vi "Calibrations Control Loop 2017.vi"   [LabVIEW 2016]
uses:
  <vilib>/Rock Robotics/Network Tables/SD Read Boolean.vi
  Global Variables/Ball Intake Calibrations.vi
  Global Variables/Deadband Calibrations.vi
  Global Variables/High Gear Calibrations.vi
  Global Variables/Low Gear Calibrations.vi
  Global Variables/Shooter Calibrations.vi
  Global Variables/Turn to Heading Calibrations.vi
  Global Variables/Drive Path Calibrations.vi
  Global Variables/Conveyor Calibrations.vi
  Global Variables/Auto Drive Calibrations.vi
  <vilib>/Rock Robotics/Network Tables/NT Write Numeric Array.vi
  <vilib>/Rock Robotics/Network Tables/NT Read Numeric Array.vi
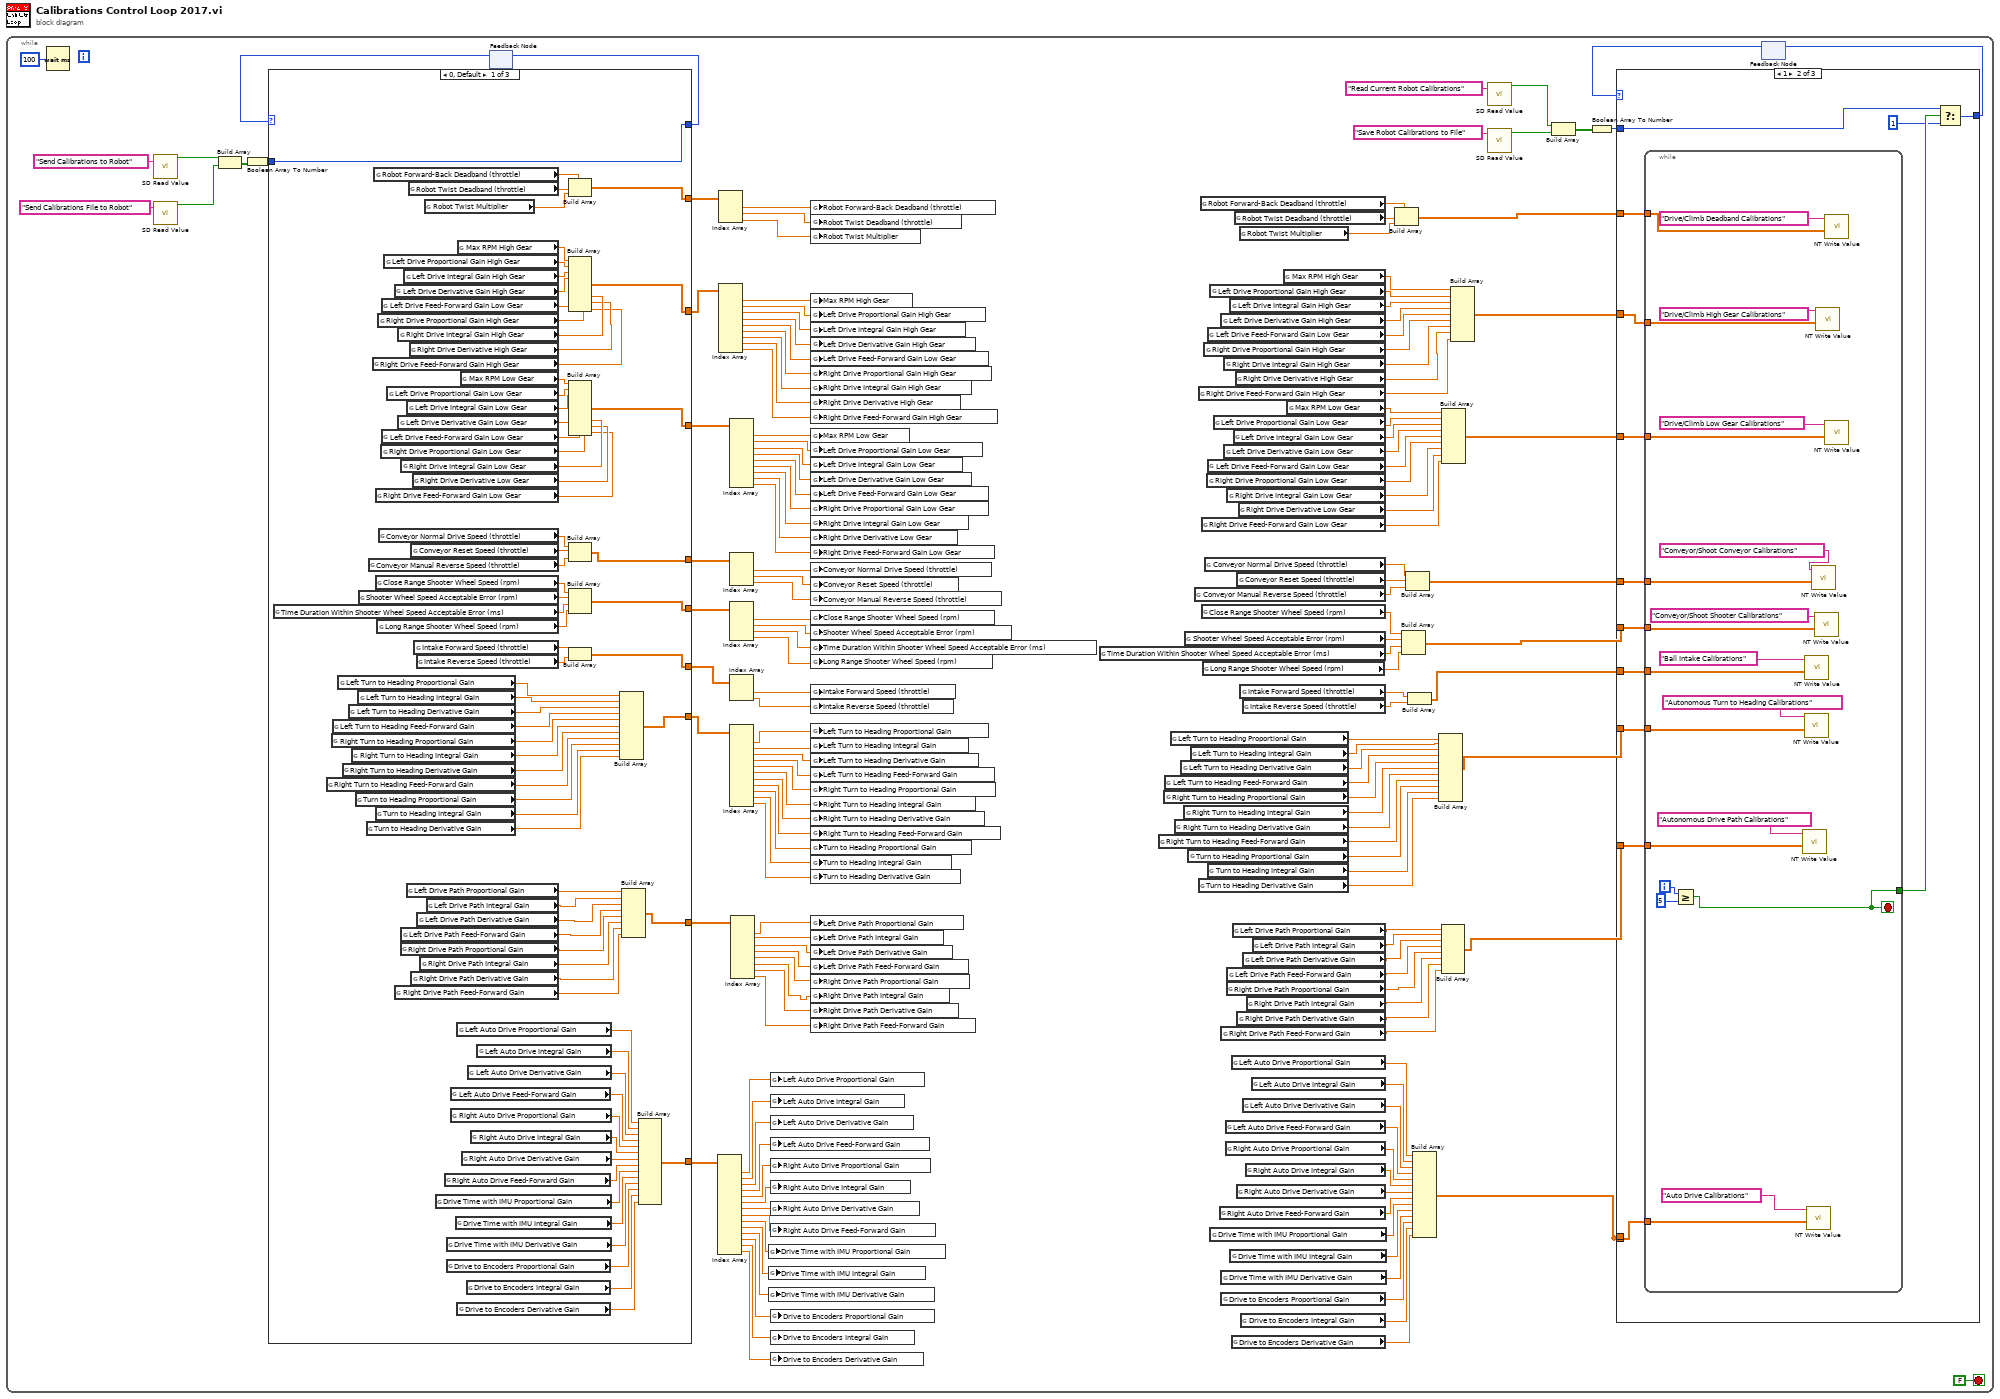
[diagram p0: block diagram]
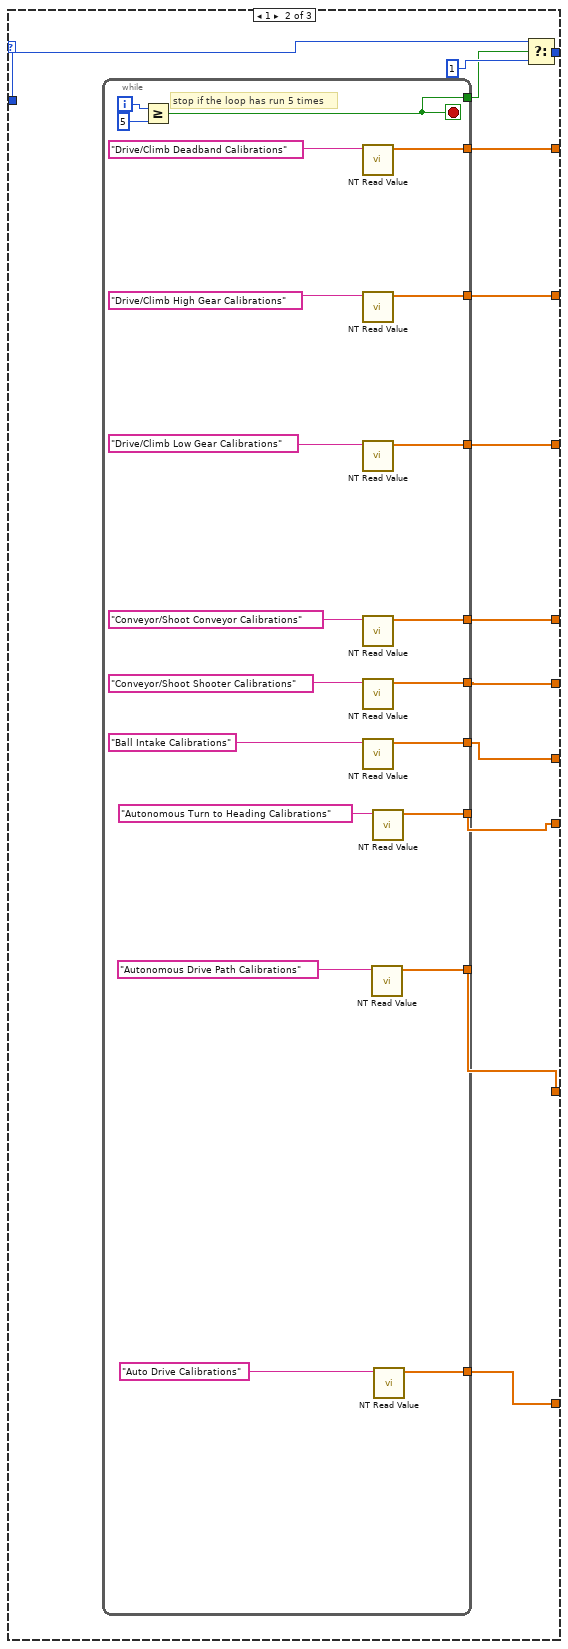
[diagram p2: hidden frame]
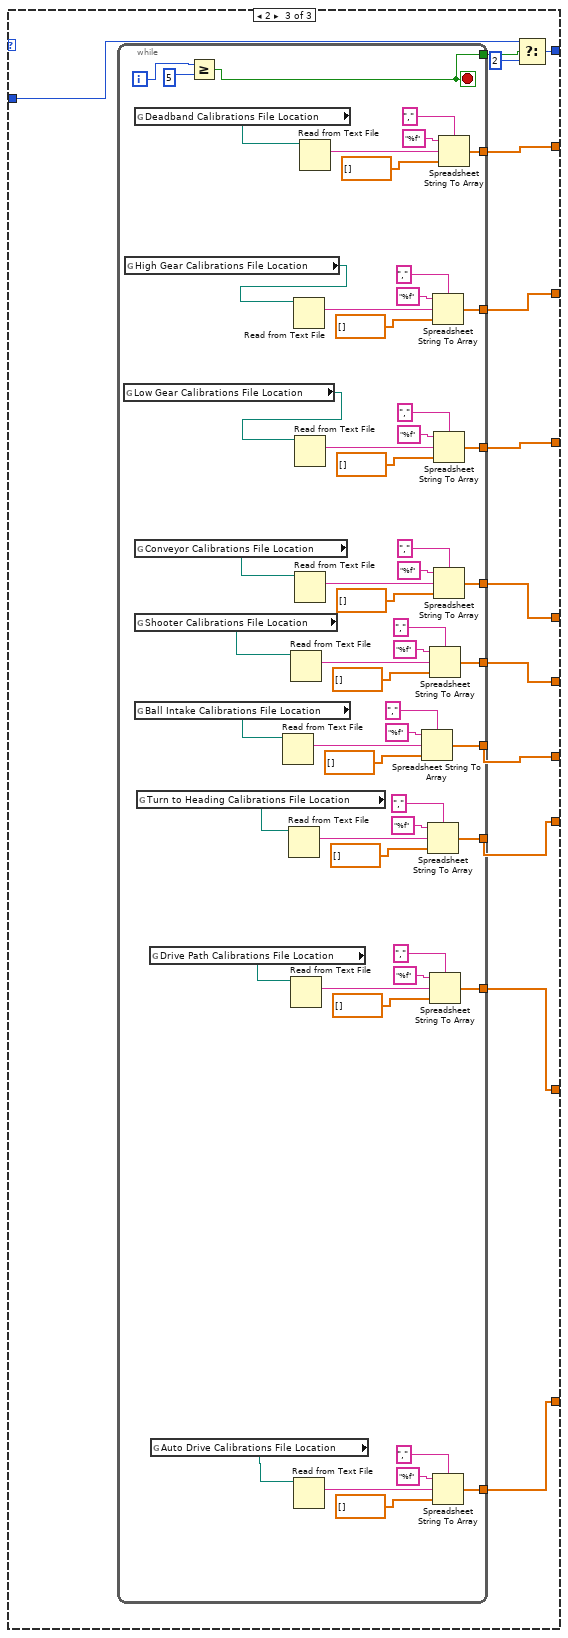
[diagram p3: hidden frame]
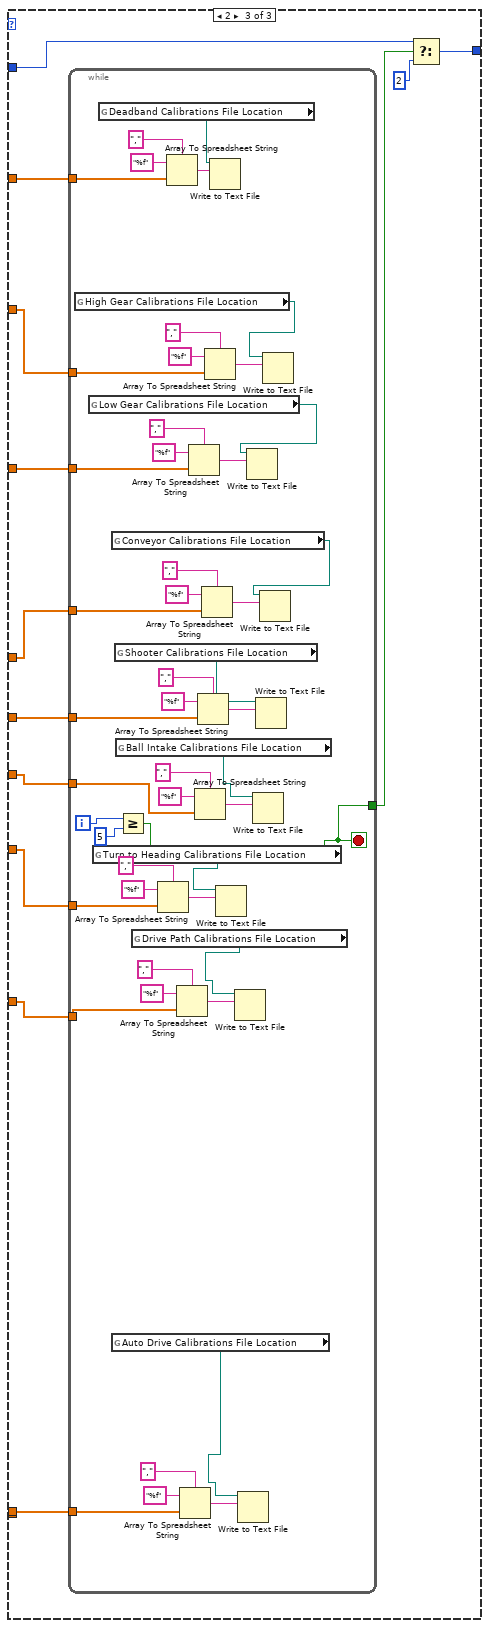
[diagram p5: hidden frame]
diagram:
  n1 = while {
    stop <- FALSE stop-if-true
    n2 = Wait (ms)(milliseconds to wait=u32 100) -> ()  [unwired: 1 out]
    n3 = call-poly <vilib>:"SD Read Value.vi"("Name"="Send Calibrations to Robot") -> ("Boolean"=w152:bool)  [unwired: 8 in, 2 out]
    n4 = call-poly <vilib>:"SD Read Value.vi"("Name"="Send Calibrations File to Robot") -> ("Boolean"=w153:bool)  [unwired: 8 in, 2 out]
    n5 = Build Array(w152, w153) -> (w151:bool[])
    n6 = Boolean Array To Number(Boolean array=w151) -> (number=w148:u32)
    n7 = feedback #1() -> (w147:u32)  [unwired: 1 in]
    n8 = case shown="0, Default" w147 {
      tunnel: [w207 w248 w282] -> w156
      tunnel: w148 -> [w235 w247 w280]
      tunnel: [w235 w245 w281] -> w146
      tunnel: [w206 w244 w278] -> w142
      tunnel: [w205 w243 w277] -> w141
      tunnel: [w204 w242 w276] -> w140
      tunnel: [w203 w241 w275] -> w133
      tunnel: [w202 w240 w274] -> w139
      tunnel: [w193 w239 w273] -> w40
      tunnel: [w184 w238 w272] -> w73
      tunnel: [w177 w236 w270] -> w30
      frame 0, Default {
        n9 = global read "Shooter Calibrations.vi" "Time Duration Within Shooter Wheel Speed Acceptable Error (ms)"() -> (w211:dbl)
        n10 = global read "Turn to Heading Calibrations.vi" "Right Turn to Heading Feed-Forward Gain"() -> (w194:dbl)
        n11 = global read "Turn to Heading Calibrations.vi" "Right Turn to Heading Proportional Gain"() -> (w197:dbl)
        n12 = global read "Turn to Heading Calibrations.vi" "Left Turn to Heading Feed-Forward Gain"() -> (w198:dbl)
        n13 = global read "Turn to Heading Calibrations.vi" "Left Turn to Heading Proportional Gain"() -> (w201:dbl)
        n14 = global read "Turn to Heading Calibrations.vi" "Right Turn to Heading Derivative Gain"() -> (w195:dbl)
        n15 = global read "Turn to Heading Calibrations.vi" "Left Turn to Heading Derivative Gain"() -> (w199:dbl)
        n16 = global read "Turn to Heading Calibrations.vi" "Right Turn to Heading Integral Gain"() -> (w196:dbl)
        n17 = global read "Turn to Heading Calibrations.vi" "Turn to Heading Proportional Gain"() -> (w181:dbl)
        n18 = global read "Turn to Heading Calibrations.vi" "Left Turn to Heading Integral Gain"() -> (w200:dbl)
        n19 = global read "Shooter Calibrations.vi" "Shooter Wheel Speed Acceptable Error (rpm)"() -> (w212:dbl)
        n20 = global read "Turn to Heading Calibrations.vi" "Turn to Heading Derivative Gain"() -> (w179:dbl)
        n21 = global read "Conveyor Calibrations.vi" "Conveyor Manual Reverse Speed (throttle)"() -> (w213:dbl)
        n22 = global read "High Gear Calibrations.vi" "Right Drive Feed-Forward Gain High Gear"() -> (w224:dbl)
        n23 = global read "Deadband Calibrations.vi" "Robot Forward-Back Deadband (throttle)"() -> (w233:dbl)
        n24 = global read "Low Gear Calibrations.vi" "Right Drive Feed-Forward Gain Low Gear"() -> (w208:dbl)
        n25 = global read "Shooter Calibrations.vi" "Close Range Shooter Wheel Speed (rpm)"() -> (w183:dbl)
        n26 = global read "Turn to Heading Calibrations.vi" "Turn to Heading Integral Gain"() -> (w180:dbl)
        n27 = global read "Shooter Calibrations.vi" "Long Range Shooter Wheel Speed (rpm)"() -> (w182:dbl)
        n28 = global read "High Gear Calibrations.vi" "Right Drive Proportional Gain High Gear"() -> (w227:dbl)
        n29 = global read "Conveyor Calibrations.vi" "Conveyor Normal Drive Speed (throttle)"() -> (w215:dbl)
        n30 = global read "Low Gear Calibrations.vi" "Right Drive Proportional Gain Low Gear"() -> (w218:dbl)
        n31 = global read "High Gear Calibrations.vi" "Left Drive Feed-Forward Gain Low Gear"() -> (w228:dbl)
        n32 = global read "Low Gear Calibrations.vi" "Left Drive Feed-Forward Gain Low Gear"() -> (w219:dbl)
        n33 = global read "High Gear Calibrations.vi" "Left Drive Proportional Gain High Gear"() -> (w231:dbl)
        n34 = global read "Low Gear Calibrations.vi" "Left Drive Proportional Gain Low Gear"() -> (w222:dbl)
        n35 = global read "High Gear Calibrations.vi" "Left Drive Derivative Gain High Gear"() -> (w229:dbl)
        n36 = global read "Drive Path Calibrations.vi" "Right Drive Path Feed-Forward Gain"() -> (w190:dbl)
        n37 = global read "High Gear Calibrations.vi" "Right Drive Integral Gain High Gear"() -> (w226:dbl)
        n38 = global read "Low Gear Calibrations.vi" "Left Drive Derivative Gain Low Gear"() -> (w220:dbl)
        n39 = global read "Drive Path Calibrations.vi" "Right Drive Path Proportional Gain"() -> (w185:dbl)
        n40 = global read "Low Gear Calibrations.vi" "Right Drive Integral Gain Low Gear"() -> (w217:dbl)
        n41 = global read "Drive Path Calibrations.vi" "Left Drive Path Feed-Forward Gain"() -> (w186:dbl)
        n42 = global read "High Gear Calibrations.vi" "Left Drive Integral Gain High Gear"() -> (w230:dbl)
        n43 = global read "Drive Path Calibrations.vi" "Left Drive Path Proportional Gain"() -> (w192:dbl)
        n44 = global read "Low Gear Calibrations.vi" "Left Drive Integral Gain Low Gear"() -> (w221:dbl)
        n45 = global read "Deadband Calibrations.vi" "Robot Twist Deadband (throttle)"() -> (w234:dbl)
        n46 = global read "High Gear Calibrations.vi" "Right Drive Derivative High Gear"() -> (w225:dbl)
        n47 = global read "Conveyor Calibrations.vi" "Conveyor Reset Speed (throttle)"() -> (w214:dbl)
        n48 = global read "Drive Path Calibrations.vi" "Right Drive Path Derivative Gain"() -> (w189:dbl)
        n49 = global read "Low Gear Calibrations.vi" "Right Drive Derivative Low Gear"() -> (w216:dbl)
        n50 = global read "Ball Intake Calibrations.vi" "Intake Forward Speed (throttle)"() -> (w210:dbl)
        n51 = global read "Ball Intake Calibrations.vi" "Intake Reverse Speed (throttle)"() -> (w209:dbl)
        n52 = global read "Drive Path Calibrations.vi" "Left Drive Path Derivative Gain"() -> (w187:dbl)
        n53 = global read "Drive Path Calibrations.vi" "Right Drive Path Integral Gain"() -> (w188:dbl)
        n54 = global read "Deadband Calibrations.vi" "Robot Twist Multiplier"() -> (w178:dbl)
        n55 = global read "Drive Path Calibrations.vi" "Left Drive Path Integral Gain"() -> (w191:dbl)
        n56 = global read "Auto Drive Calibrations.vi" "Drive Time with IMU Proportional Gain"() -> (w168:dbl)
        n57 = global read "Auto Drive Calibrations.vi" "Right Auto Drive Feed-Forward Gain"() -> (w169:dbl)
        n58 = global read "Auto Drive Calibrations.vi" "Drive Time with IMU Derivative Gain"() -> (w166:dbl)
        n59 = global read "Auto Drive Calibrations.vi" "Drive to Encoders Proportional Gain"() -> (w165:dbl)
        n60 = global read "Auto Drive Calibrations.vi" "Left Auto Drive Feed-Forward Gain"() -> (w173:dbl)
        n61 = global read "Auto Drive Calibrations.vi" "Right Auto Drive Proportional Gain"() -> (w172:dbl)
        n62 = global read "Auto Drive Calibrations.vi" "Drive Time with IMU Integral Gain"() -> (w167:dbl)
        n63 = global read "Auto Drive Calibrations.vi" "Left Auto Drive Proportional Gain"() -> (w176:dbl)
        n64 = global read "Auto Drive Calibrations.vi" "Drive to Encoders Derivative Gain"() -> (w163:dbl)
        n65 = global read "High Gear Calibrations.vi" "Max RPM High Gear"() -> (w232:dbl)
        n66 = global read "Low Gear Calibrations.vi" "Max RPM Low Gear"() -> (w223:dbl)
        n67 = global read "Auto Drive Calibrations.vi" "Right Auto Drive Derivative Gain"() -> (w170:dbl)
        n68 = global read "Auto Drive Calibrations.vi" "Drive to Encoders Integral Gain"() -> (w164:dbl)
        n69 = global read "Auto Drive Calibrations.vi" "Left Auto Drive Derivative Gain"() -> (w174:dbl)
        n70 = global read "Auto Drive Calibrations.vi" "Right Auto Drive Integral Gain"() -> (w171:dbl)
        n71 = global read "Auto Drive Calibrations.vi" "Left Auto Drive Integral Gain"() -> (w175:dbl)
        n72 = Build Array(w233, w234, w178) -> (w207:dbl[])
        n73 = Build Array(w232, w231, w230, w229, w228, w227, w226, w225, w224) -> (w206:dbl[])
        n74 = Build Array(w223, w222, w221, w220, w219, w218, w217, w216, w208) -> (w205:dbl[])
        n75 = Build Array(w215, w214, w213) -> (w204:dbl[])
        n76 = Build Array(w183, w212, w211, w182) -> (w203:dbl[])
        n77 = Build Array(w210, w209) -> (w202:dbl[])
        n78 = Build Array(w201, w200, w199, w198, w197, w196, w195, w194, w181, w180, w179) -> (w193:dbl[])
        n79 = Build Array(w192, w191, w187, w186, w185, w188, w189, w190) -> (w184:dbl[])
        n80 = Build Array(w176, w175, w174, w173, w172, w171, w170, w169, w168, w167, w166, w165, w164, w163) -> (w177:dbl[])
      }
      frame 1 {
        n81 = while {
          tunnel: [w269] -> w248
          tunnel: [w265] -> w237
          tunnel: [w259] -> w244
          tunnel: [w258] -> w243
          tunnel: [w257] -> w242
          tunnel: [w256] -> w241
          tunnel: [w255] -> w240
          tunnel: [w253] -> w239
          tunnel: [w251] -> w238
          tunnel: [w249] -> w236
          i -> [w267]
          stop <- w265 stop-if-true
          # "stop if the loop has run 5 times"
          n82 = Greater Or Equal?(x=w267, y=5) -> (x >= y?=w265:bool)
          n83 = call-poly <vilib>:"NT Read Value.vi"("Name"="Drive/Climb Deadband Calibrations") -> ("Numeric Array"=w269:dbl[])  [unwired: 9 in, 1 out]
          n84 = call-poly <vilib>:"NT Read Value.vi"("Name"="Drive/Climb High Gear Calibrations") -> ("Numeric Array"=w259:dbl[])  [unwired: 9 in, 1 out]
          n85 = call-poly <vilib>:"NT Read Value.vi"("Name"="Drive/Climb Low Gear Calibrations") -> ("Numeric Array"=w258:dbl[])  [unwired: 9 in, 1 out]
          n86 = call-poly <vilib>:"NT Read Value.vi"("Name"="Conveyor/Shoot Conveyor Calibrations") -> ("Numeric Array"=w257:dbl[])  [unwired: 9 in, 1 out]
          n87 = call-poly <vilib>:"NT Read Value.vi"("Name"="Conveyor/Shoot Shooter Calibrations") -> ("Numeric Array"=w256:dbl[])  [unwired: 9 in, 1 out]
          n88 = call-poly <vilib>:"NT Read Value.vi"("Name"="Ball Intake Calibrations") -> ("Numeric Array"=w255:dbl[])  [unwired: 9 in, 1 out]
          n89 = call-poly <vilib>:"NT Read Value.vi"("Name"="Autonomous Drive Path Calibrations") -> ("Numeric Array"=w251:dbl[])  [unwired: 9 in, 1 out]
          n90 = call-poly <vilib>:"NT Read Value.vi"("Name"="Autonomous Turn to Heading Calibrations") -> ("Numeric Array"=w253:dbl[])  [unwired: 9 in, 1 out]
          n91 = call-poly <vilib>:"NT Read Value.vi"("Name"="Auto Drive Calibrations") -> ("Numeric Array"=w249:dbl[])  [unwired: 9 in, 1 out]
        }
        n92 = Select(t=w247, s=w237, f=1) -> (s? t:f=w245:u32)
      }
      frame 2 {
        n93 = while {
          tunnel: [w339] -> w282
          tunnel: [w338] -> w278
          tunnel: [w337] -> w277
          tunnel: [w336] -> w276
          tunnel: [w335] -> w275
          tunnel: [w334] -> w274
          tunnel: [w295] -> w272
          tunnel: [w293] -> w273
          tunnel: [w289] -> w271
          tunnel: [w283] -> w270
          i -> [w305]
          stop <- w289 stop-if-true
          n94 = global read "Low Gear Calibrations.vi" "Low Gear Calibrations File Location"() -> (w291:path)
          n95 = global read "High Gear Calibrations.vi" "High Gear Calibrations File Location"() -> (w292:path)
          n96 = global read "Deadband Calibrations.vi" "Deadband Calibrations File Location"() -> (w329:path)
          n97 = global read "Conveyor Calibrations.vi" "Conveyor Calibrations File Location"() -> (w308:path)
          n98 = global read "Shooter Calibrations.vi" "Shooter Calibrations File Location"() -> (w307:path)
          n99 = global read "Ball Intake Calibrations.vi" "Ball Intake Calibrations File Location"() -> (w306:path)
          n100 = global read "Turn to Heading Calibrations.vi" "Turn to Heading Calibrations File Location"() -> (w294:path)
          n101 = global read "Drive Path Calibrations.vi" "Drive Path Calibrations File Location"() -> (w290:path)
          n102 = global read "Auto Drive Calibrations.vi" "Auto Drive Calibrations File Location"() -> (w284:path)
          n103 = Greater Or Equal?(x=w305, y=5) -> (x >= y?=w289:bool)
          n104 = Read from Text File(file (use dialog)=w306) -> (text=w312:string)  [unwired: 3 in, 3 out]
          n105 = Read from Text File(file (use dialog)=w294) -> (text=w303:string)  [unwired: 3 in, 3 out]
          n106 = Read from Text File(file (use dialog)=w307) -> (text=w316:string)  [unwired: 3 in, 3 out]
          n107 = Read from Text File(file (use dialog)=w290) -> (text=w299:string)  [unwired: 3 in, 3 out]
          n108 = Read from Text File(file (use dialog)=w292) -> (text=w328:string)  [unwired: 3 in, 3 out]
          n109 = Read from Text File(file (use dialog)=w284) -> (text=w288:string)  [unwired: 3 in, 3 out]
          n110 = Read from Text File(file (use dialog)=w291) -> (text=w324:string)  [unwired: 3 in, 3 out]
          n111 = Read from Text File(file (use dialog)=w308) -> (text=w320:string)  [unwired: 3 in, 3 out]
          n112 = Read from Text File(file (use dialog)=w329) -> (text=w333:string)  [unwired: 3 in, 3 out]
          n113 = Spreadsheet String To Array(delimiter (Tab)=",", format string="%f", spreadsheet string=w312, array type (2D Dbl)=dbl[] []) -> (array=w334:dbl[])
          n114 = Spreadsheet String To Array(delimiter (Tab)=",", format string="%f", spreadsheet string=w303, array type (2D Dbl)=dbl[] []) -> (array=w293:dbl[])
          n115 = Spreadsheet String To Array(delimiter (Tab)=",", format string="%f", spreadsheet string=w316, array type (2D Dbl)=dbl[] []) -> (array=w335:dbl[])
          n116 = Spreadsheet String To Array(delimiter (Tab)=",", format string="%f", spreadsheet string=w299, array type (2D Dbl)=dbl[] []) -> (array=w295:dbl[])
          n117 = Spreadsheet String To Array(delimiter (Tab)=",", format string="%f", spreadsheet string=w328, array type (2D Dbl)=dbl[] []) -> (array=w338:dbl[])
          n118 = Spreadsheet String To Array(delimiter (Tab)=",", format string="%f", spreadsheet string=w288, array type (2D Dbl)=dbl[] []) -> (array=w283:dbl[])
          n119 = Spreadsheet String To Array(delimiter (Tab)=",", format string="%f", spreadsheet string=w324, array type (2D Dbl)=dbl[] []) -> (array=w337:dbl[])
          n120 = Spreadsheet String To Array(delimiter (Tab)=",", format string="%f", spreadsheet string=w320, array type (2D Dbl)=dbl[] []) -> (array=w336:dbl[])
          n121 = Spreadsheet String To Array(delimiter (Tab)=",", format string="%f", spreadsheet string=w333, array type (2D Dbl)=dbl[] []) -> (array=w339:dbl[])
        }
        n122 = Select(t=w280, s=w271, f=u32 2) -> (s? t:f=w281:u32)
      }
    }
    n123 = feedback-in #1(w146) -> ()
    n124 = Index Array(array=w30) -> (element #1=w29:dbl, element #2=w28:dbl, element #3=w27:dbl, element #4=w26:dbl, element #5=w25:dbl, element #6=w24:dbl, element #7=w23:dbl, element #8=w22:dbl, element #9=w21:dbl, element #10=w20:dbl, element #11=w19:dbl, element #12=w18:dbl, element #13=w17:dbl, element #14=w16:dbl)  [unwired: 14 in]
    n125 = Index Array(array=w156) -> (element #1=w132:dbl, element #2=w131:dbl, element #3=w32:dbl)  [unwired: 3 in]
    n126 = Index Array(array=w142) -> (element #1=w127:dbl, element #2=w100:dbl, element #3=w99:dbl, element #4=w98:dbl, element #5=w97:dbl, element #6=w96:dbl, element #7=w95:dbl, element #8=w94:dbl, element #9=w93:dbl)  [unwired: 9 in]
    n127 = Index Array(array=w141) -> (element #1=w128:dbl, element #2=w92:dbl, element #3=w91:dbl, element #4=w90:dbl, element #5=w89:dbl, element #6=w88:dbl, element #7=w87:dbl, element #8=w86:dbl, element #9=w85:dbl)  [unwired: 9 in]
    n128 = Index Array(array=w140) -> (element #1=w84:dbl, element #2=w83:dbl, element #3=w129:dbl)  [unwired: 3 in]
    n129 = Index Array(array=w133) -> (element #1=w44:dbl, element #2=w42:dbl, element #3=w41:dbl, element #4=w43:dbl)  [unwired: 4 in]
    n130 = Index Array(array=w139) -> (element #1=w130:dbl, element #2=w82:dbl)  [unwired: 2 in]
    n131 = Index Array(array=w40) -> (element #1=w81:dbl, element #2=w80:dbl, element #3=w79:dbl, element #4=w78:dbl, element #5=w77:dbl, element #6=w76:dbl, element #7=w75:dbl, element #8=w74:dbl, element #9=w39:dbl, element #10=w38:dbl, element #11=w37:dbl)  [unwired: 11 in]
    n132 = Index Array(array=w73) -> (element #1=w72:dbl, element #2=w71:dbl, element #3=w70:dbl, element #4=w69:dbl, element #5=w68:dbl, element #6=w67:dbl, element #7=w66:dbl, element #8=w65:dbl)  [unwired: 8 in]
    n133 = global write "Auto Drive Calibrations.vi" "Drive Time with IMU Proportional Gain"(w21) -> ()
    n134 = global write "Auto Drive Calibrations.vi" "Drive Time with IMU Integral Gain"(w20) -> ()
    n135 = global write "Auto Drive Calibrations.vi" "Drive Time with IMU Derivative Gain"(w19) -> ()
    n136 = global write "Auto Drive Calibrations.vi" "Left Auto Drive Proportional Gain"(w29) -> ()
    n137 = global write "Auto Drive Calibrations.vi" "Left Auto Drive Integral Gain"(w28) -> ()
    n138 = global write "Auto Drive Calibrations.vi" "Left Auto Drive Derivative Gain"(w27) -> ()
    n139 = global write "Auto Drive Calibrations.vi" "Left Auto Drive Feed-Forward Gain"(w26) -> ()
    n140 = global write "Auto Drive Calibrations.vi" "Right Auto Drive Proportional Gain"(w25) -> ()
    n141 = global write "Auto Drive Calibrations.vi" "Right Auto Drive Integral Gain"(w24) -> ()
    n142 = global write "Auto Drive Calibrations.vi" "Right Auto Drive Derivative Gain"(w23) -> ()
    n143 = global write "Auto Drive Calibrations.vi" "Right Auto Drive Feed-Forward Gain"(w22) -> ()
    n144 = global write "Auto Drive Calibrations.vi" "Drive to Encoders Proportional Gain"(w18) -> ()
    n145 = global write "Auto Drive Calibrations.vi" "Drive to Encoders Integral Gain"(w17) -> ()
    n146 = global write "Auto Drive Calibrations.vi" "Drive to Encoders Derivative Gain"(w16) -> ()
    n147 = global write "Deadband Calibrations.vi" "Robot Forward-Back Deadband (throttle)"(w132) -> ()
    n148 = global write "Deadband Calibrations.vi" "Robot Twist Deadband (throttle)"(w131) -> ()
    n149 = global write "Deadband Calibrations.vi" "Robot Twist Multiplier"(w32) -> ()
    n150 = global write "High Gear Calibrations.vi" "Max RPM High Gear"(w127) -> ()
    n151 = global write "High Gear Calibrations.vi" "Left Drive Proportional Gain High Gear"(w100) -> ()
    n152 = global write "High Gear Calibrations.vi" "Left Drive Integral Gain High Gear"(w99) -> ()
    n153 = global write "High Gear Calibrations.vi" "Left Drive Derivative Gain High Gear"(w98) -> ()
    n154 = global write "High Gear Calibrations.vi" "Left Drive Feed-Forward Gain Low Gear"(w97) -> ()
    n155 = global write "High Gear Calibrations.vi" "Right Drive Proportional Gain High Gear"(w96) -> ()
    n156 = global write "High Gear Calibrations.vi" "Right Drive Integral Gain High Gear"(w95) -> ()
    n157 = global write "High Gear Calibrations.vi" "Right Drive Derivative High Gear"(w94) -> ()
    n158 = global write "High Gear Calibrations.vi" "Right Drive Feed-Forward Gain High Gear"(w93) -> ()
    n159 = global write "Low Gear Calibrations.vi" "Max RPM Low Gear"(w128) -> ()
    n160 = global write "Low Gear Calibrations.vi" "Left Drive Proportional Gain Low Gear"(w92) -> ()
    n161 = global write "Low Gear Calibrations.vi" "Left Drive Integral Gain Low Gear"(w91) -> ()
    n162 = global write "Low Gear Calibrations.vi" "Left Drive Derivative Gain Low Gear"(w90) -> ()
    n163 = global write "Low Gear Calibrations.vi" "Left Drive Feed-Forward Gain Low Gear"(w89) -> ()
    n164 = global write "Low Gear Calibrations.vi" "Right Drive Proportional Gain Low Gear"(w88) -> ()
    n165 = global write "Low Gear Calibrations.vi" "Right Drive Integral Gain Low Gear"(w87) -> ()
    n166 = global write "Low Gear Calibrations.vi" "Right Drive Derivative Low Gear"(w86) -> ()
    n167 = global write "Low Gear Calibrations.vi" "Right Drive Feed-Forward Gain Low Gear"(w85) -> ()
    n168 = global write "Conveyor Calibrations.vi" "Conveyor Normal Drive Speed (throttle)"(w84) -> ()
    n169 = global write "Conveyor Calibrations.vi" "Conveyor Reset Speed (throttle)"(w83) -> ()
    n170 = global write "Conveyor Calibrations.vi" "Conveyor Manual Reverse Speed (throttle)"(w129) -> ()
    n171 = global write "Shooter Calibrations.vi" "Close Range Shooter Wheel Speed (rpm)"(w44) -> ()
    n172 = global write "Shooter Calibrations.vi" "Shooter Wheel Speed Acceptable Error (rpm)"(w42) -> ()
    n173 = global write "Shooter Calibrations.vi" "Time Duration Within Shooter Wheel Speed Acceptable Error (ms)"(w41) -> ()
    n174 = global write "Shooter Calibrations.vi" "Long Range Shooter Wheel Speed (rpm)"(w43) -> ()
    n175 = global write "Ball Intake Calibrations.vi" "Intake Forward Speed (throttle)"(w130) -> ()
    n176 = global write "Ball Intake Calibrations.vi" "Intake Reverse Speed (throttle)"(w82) -> ()
    n177 = global write "Turn to Heading Calibrations.vi" "Left Turn to Heading Proportional Gain"(w81) -> ()
    n178 = global write "Turn to Heading Calibrations.vi" "Left Turn to Heading Integral Gain"(w80) -> ()
    n179 = global write "Turn to Heading Calibrations.vi" "Left Turn to Heading Derivative Gain"(w79) -> ()
    n180 = global write "Turn to Heading Calibrations.vi" "Left Turn to Heading Feed-Forward Gain"(w78) -> ()
    n181 = global write "Turn to Heading Calibrations.vi" "Right Turn to Heading Proportional Gain"(w77) -> ()
    n182 = global write "Turn to Heading Calibrations.vi" "Right Turn to Heading Integral Gain"(w76) -> ()
    n183 = global write "Turn to Heading Calibrations.vi" "Right Turn to Heading Derivative Gain"(w75) -> ()
    n184 = global write "Turn to Heading Calibrations.vi" "Right Turn to Heading Feed-Forward Gain"(w74) -> ()
    n185 = global write "Turn to Heading Calibrations.vi" "Turn to Heading Proportional Gain"(w39) -> ()
    n186 = global write "Turn to Heading Calibrations.vi" "Turn to Heading Integral Gain"(w38) -> ()
    n187 = global write "Turn to Heading Calibrations.vi" "Turn to Heading Derivative Gain"(w37) -> ()
    n188 = global write "Drive Path Calibrations.vi" "Left Drive Path Proportional Gain"(w72) -> ()
    n189 = global write "Drive Path Calibrations.vi" "Left Drive Path Integral Gain"(w71) -> ()
    n190 = global write "Drive Path Calibrations.vi" "Left Drive Path Derivative Gain"(w70) -> ()
    n191 = global write "Drive Path Calibrations.vi" "Left Drive Path Feed-Forward Gain"(w69) -> ()
    n192 = global write "Drive Path Calibrations.vi" "Right Drive Path Proportional Gain"(w68) -> ()
    n193 = global write "Drive Path Calibrations.vi" "Right Drive Path Integral Gain"(w67) -> ()
    n194 = global write "Drive Path Calibrations.vi" "Right Drive Path Derivative Gain"(w66) -> ()
    n195 = global write "Drive Path Calibrations.vi" "Right Drive Path Feed-Forward Gain"(w65) -> ()
    n196 = global read "Shooter Calibrations.vi" "Time Duration Within Shooter Wheel Speed Acceptable Error (ms)"() -> (w104:dbl)
    n197 = global read "Turn to Heading Calibrations.vi" "Right Turn to Heading Feed-Forward Gain"() -> (w58:dbl)
    n198 = global read "Turn to Heading Calibrations.vi" "Right Turn to Heading Proportional Gain"() -> (w61:dbl)
    n199 = global read "Turn to Heading Calibrations.vi" "Left Turn to Heading Feed-Forward Gain"() -> (w62:dbl)
    n200 = global read "Turn to Heading Calibrations.vi" "Left Turn to Heading Proportional Gain"() -> (w64:dbl)
    n201 = global read "Turn to Heading Calibrations.vi" "Right Turn to Heading Derivative Gain"() -> (w59:dbl)
    n202 = global read "Turn to Heading Calibrations.vi" "Left Turn to Heading Derivative Gain"() -> (w63:dbl)
    n203 = global read "Turn to Heading Calibrations.vi" "Right Turn to Heading Integral Gain"() -> (w60:dbl)
    n204 = global read "Shooter Calibrations.vi" "Shooter Wheel Speed Acceptable Error (rpm)"() -> (w105:dbl)
    n205 = global read "Turn to Heading Calibrations.vi" "Turn to Heading Proportional Gain"() -> (w35:dbl)
    n206 = global read "Turn to Heading Calibrations.vi" "Left Turn to Heading Integral Gain"() -> (w36:dbl)
    n207 = global read "Conveyor Calibrations.vi" "Conveyor Manual Reverse Speed (throttle)"() -> (w106:dbl)
    n208 = global read "High Gear Calibrations.vi" "Right Drive Feed-Forward Gain High Gear"() -> (w116:dbl)
    n209 = global read "Turn to Heading Calibrations.vi" "Turn to Heading Derivative Gain"() -> (w33:dbl)
    n210 = global read "Deadband Calibrations.vi" "Robot Forward-Back Deadband (throttle)"() -> (w125:dbl)
    n211 = global read "Low Gear Calibrations.vi" "Right Drive Feed-Forward Gain Low Gear"() -> (w101:dbl)
    n212 = global read "Shooter Calibrations.vi" "Close Range Shooter Wheel Speed (rpm)"() -> (w45:dbl)
    n213 = global read "Shooter Calibrations.vi" "Long Range Shooter Wheel Speed (rpm)"() -> (w46:dbl)
    n214 = global read "High Gear Calibrations.vi" "Right Drive Proportional Gain High Gear"() -> (w119:dbl)
    n215 = global read "Conveyor Calibrations.vi" "Conveyor Normal Drive Speed (throttle)"() -> (w47:dbl)
    n216 = global read "Low Gear Calibrations.vi" "Right Drive Proportional Gain Low Gear"() -> (w110:dbl)
    n217 = global read "High Gear Calibrations.vi" "Left Drive Feed-Forward Gain Low Gear"() -> (w120:dbl)
    n218 = global read "Low Gear Calibrations.vi" "Left Drive Feed-Forward Gain Low Gear"() -> (w111:dbl)
    n219 = global read "Turn to Heading Calibrations.vi" "Turn to Heading Integral Gain"() -> (w34:dbl)
    n220 = global read "High Gear Calibrations.vi" "Left Drive Proportional Gain High Gear"() -> (w123:dbl)
    n221 = global read "Auto Drive Calibrations.vi" "Drive Time with IMU Proportional Gain"() -> (w7:dbl)
    n222 = global read "Low Gear Calibrations.vi" "Left Drive Proportional Gain Low Gear"() -> (w114:dbl)
    n223 = global read "Auto Drive Calibrations.vi" "Right Auto Drive Feed-Forward Gain"() -> (w8:dbl)
    n224 = global read "High Gear Calibrations.vi" "Left Drive Derivative Gain High Gear"() -> (w121:dbl)
    n225 = global read "Drive Path Calibrations.vi" "Right Drive Path Feed-Forward Gain"() -> (w50:dbl)
    n226 = global read "Auto Drive Calibrations.vi" "Drive Time with IMU Derivative Gain"() -> (w5:dbl)
    n227 = global read "Auto Drive Calibrations.vi" "Drive to Encoders Proportional Gain"() -> (w4:dbl)
    n228 = global read "High Gear Calibrations.vi" "Right Drive Integral Gain High Gear"() -> (w118:dbl)
    n229 = global read "Low Gear Calibrations.vi" "Left Drive Derivative Gain Low Gear"() -> (w112:dbl)
    n230 = global read "Auto Drive Calibrations.vi" "Left Auto Drive Feed-Forward Gain"() -> (w12:dbl)
    n231 = global read "Auto Drive Calibrations.vi" "Right Auto Drive Proportional Gain"() -> (w11:dbl)
    n232 = global read "Drive Path Calibrations.vi" "Right Drive Path Proportional Gain"() -> (w53:dbl)
    n233 = global read "Low Gear Calibrations.vi" "Right Drive Integral Gain Low Gear"() -> (w109:dbl)
    n234 = global read "Drive Path Calibrations.vi" "Left Drive Path Feed-Forward Gain"() -> (w54:dbl)
    n235 = global read "High Gear Calibrations.vi" "Left Drive Integral Gain High Gear"() -> (w122:dbl)
    n236 = global read "Auto Drive Calibrations.vi" "Drive Time with IMU Integral Gain"() -> (w6:dbl)
    n237 = global read "Auto Drive Calibrations.vi" "Left Auto Drive Proportional Gain"() -> (w15:dbl)
    n238 = global read "Auto Drive Calibrations.vi" "Drive to Encoders Derivative Gain"() -> (w2:dbl)
    n239 = global read "Drive Path Calibrations.vi" "Left Drive Path Proportional Gain"() -> (w57:dbl)
    n240 = global read "Low Gear Calibrations.vi" "Left Drive Integral Gain Low Gear"() -> (w113:dbl)
    n241 = global read "Deadband Calibrations.vi" "Robot Twist Deadband (throttle)"() -> (w126:dbl)
    n242 = global read "High Gear Calibrations.vi" "Right Drive Derivative High Gear"() -> (w117:dbl)
    n243 = global read "Auto Drive Calibrations.vi" "Right Auto Drive Derivative Gain"() -> (w9:dbl)
    n244 = global read "Conveyor Calibrations.vi" "Conveyor Reset Speed (throttle)"() -> (w107:dbl)
    n245 = global read "Drive Path Calibrations.vi" "Right Drive Path Derivative Gain"() -> (w51:dbl)
    n246 = global read "Low Gear Calibrations.vi" "Right Drive Derivative Low Gear"() -> (w108:dbl)
    n247 = global read "Deadband Calibrations.vi" "Robot Twist Multiplier"() -> (w31:dbl)
    n248 = global read "Ball Intake Calibrations.vi" "Intake Forward Speed (throttle)"() -> (w103:dbl)
    n249 = global read "Auto Drive Calibrations.vi" "Drive to Encoders Integral Gain"() -> (w3:dbl)
    n250 = global read "Ball Intake Calibrations.vi" "Intake Reverse Speed (throttle)"() -> (w102:dbl)
    n251 = global read "Auto Drive Calibrations.vi" "Left Auto Drive Derivative Gain"() -> (w13:dbl)
    n252 = global read "Drive Path Calibrations.vi" "Left Drive Path Derivative Gain"() -> (w55:dbl)
    n253 = global read "Auto Drive Calibrations.vi" "Right Auto Drive Integral Gain"() -> (w10:dbl)
    n254 = global read "Drive Path Calibrations.vi" "Right Drive Path Integral Gain"() -> (w52:dbl)
    n255 = global read "Auto Drive Calibrations.vi" "Left Auto Drive Integral Gain"() -> (w14:dbl)
    n256 = global read "Drive Path Calibrations.vi" "Left Drive Path Integral Gain"() -> (w56:dbl)
    n257 = global read "High Gear Calibrations.vi" "Max RPM High Gear"() -> (w124:dbl)
    n258 = global read "Low Gear Calibrations.vi" "Max RPM Low Gear"() -> (w115:dbl)
    n259 = Build Array(w125, w126, w31) -> (w162:dbl[])
    n260 = Build Array(w45, w105, w104, w46) -> (w135:dbl[])
    n261 = Build Array(w47, w107, w106) -> (w136:dbl[])
    n262 = Build Array(w103, w102) -> (w134:dbl[])
    n263 = Build Array(w15, w14, w13, w12, w11, w10, w9, w8, w7, w6, w5, w4, w3, w2) -> (w1:dbl[])
    n264 = Build Array(w64, w36, w63, w62, w61, w60, w59, w58, w35, w34, w33) -> (w49:dbl[])
    n265 = Build Array(w57, w56, w55, w54, w53, w52, w51, w50) -> (w48:dbl[])
    n266 = Build Array(w115, w114, w113, w112, w111, w110, w109, w108, w101) -> (w137:dbl[])
    n267 = Build Array(w124, w123, w122, w121, w120, w119, w118, w117, w116) -> (w138:dbl[])
    n268 = call-poly <vilib>:"SD Read Value.vi"("Name"="Read Current Robot Calibrations") -> ("Boolean"=w159:bool)  [unwired: 8 in, 2 out]
    n269 = call-poly <vilib>:"SD Read Value.vi"("Name"="Save Robot Calibrations to File") -> ("Boolean"=w158:bool)  [unwired: 8 in, 2 out]
    n270 = Build Array(w159, w158) -> (w157:bool[])
    n271 = Boolean Array To Number(Boolean array=w157) -> (number=w143:u32)
    n272 = feedback #2() -> (w144:u32)  [unwired: 1 in]
    n273 = case shown="1" w144 {
      tunnel: w162 -> [_ w353 w387]
      tunnel: [w340 w351 w383] -> w145
      tunnel: w143 -> [w340 w350 w386]
      tunnel: w138 -> [_ w348 w382]
      tunnel: w137 -> [_ w347 w381]
      tunnel: w136 -> [_ w346 w378]
      tunnel: w135 -> [_ w344 w379]
      tunnel: w134 -> [_ w345 w380]
      tunnel: w49 -> [_ w343 w376]
      tunnel: w48 -> [_ w342 w377]
      tunnel: w1 -> [_ w341 _]
      tunnel: w1 -> [_ _ w375]
      frame 0, Default {
      }
      frame 1 {
        n274 = while {
          tunnel: w353 -> [w366]
          tunnel: [w372] -> w352
          tunnel: w348 -> [w365]
          tunnel: w347 -> [w364]
          tunnel: w346 -> [w363]
          tunnel: w345 -> [w362]
          tunnel: w344 -> [w361]
          tunnel: w343 -> [w359]
          tunnel: w342 -> [w358]
          tunnel: w341 -> [w354]
          i -> [w374]
          stop <- w372 stop-if-true
          n275 = Greater Or Equal?(x=w374, y=5) -> (x >= y?=w372:bool)
          n276 = call-poly <vilib>:"NT Write Value.vi"("Numeric Array"=w358, "Name"="Autonomous Drive Path Calibrations") -> ()  [unwired: 9 in, 1 out]
          n277 = call-poly <vilib>:"NT Write Value.vi"("Numeric Array"=w359, "Name"="Autonomous Turn to Heading Calibrations") -> ()  [unwired: 9 in, 1 out]
          n278 = call-poly <vilib>:"NT Write Value.vi"("Numeric Array"=w362, "Name"="Ball Intake Calibrations") -> ()  [unwired: 9 in, 1 out]
          n279 = call-poly <vilib>:"NT Write Value.vi"("Numeric Array"=w354, "Name"="Auto Drive Calibrations") -> ()  [unwired: 9 in, 1 out]
          n280 = call-poly <vilib>:"NT Write Value.vi"("Numeric Array"=w363, "Name"="Conveyor/Shoot Conveyor Calibrations") -> ()  [unwired: 9 in, 1 out]
          n281 = call-poly <vilib>:"NT Write Value.vi"("Numeric Array"=w361, "Name"="Conveyor/Shoot Shooter Calibrations") -> ()  [unwired: 9 in, 1 out]
          n282 = call-poly <vilib>:"NT Write Value.vi"("Numeric Array"=w365, "Name"="Drive/Climb High Gear Calibrations") -> ()  [unwired: 9 in, 1 out]
          n283 = call-poly <vilib>:"NT Write Value.vi"("Numeric Array"=w366, "Name"="Drive/Climb Deadband Calibrations") -> ()  [unwired: 9 in, 1 out]
          n284 = call-poly <vilib>:"NT Write Value.vi"("Numeric Array"=w364, "Name"="Drive/Climb Low Gear Calibrations") -> ()  [unwired: 9 in, 1 out]
        }
        n285 = Select(t=w350, s=w352, f=u32 1) -> (s? t:f=w351:u32)
      }
      frame 2 {
        n286 = while {
          tunnel: w387 -> [w410]
          tunnel: [w430] -> w385
          tunnel: w382 -> [w409]
          tunnel: w381 -> [w408]
          tunnel: w380 -> [w407]
          tunnel: w379 -> [w406]
          tunnel: w378 -> [w405]
          tunnel: w377 -> [w400]
          tunnel: w376 -> [w395]
          tunnel: w375 -> [w388]
          i -> [w432]
          stop <- w430 stop-if-true
          n287 = global read "High Gear Calibrations.vi" "High Gear Calibrations File Location"() -> (w393:path)
          n288 = global read "Low Gear Calibrations.vi" "Low Gear Calibrations File Location"() -> (w394:path)
          n289 = global read "Turn to Heading Calibrations.vi" "Turn to Heading Calibrations File Location"() -> (w396:path)
          n290 = global read "Deadband Calibrations.vi" "Deadband Calibrations File Location"() -> (w429:path)
          n291 = global read "Conveyor Calibrations.vi" "Conveyor Calibrations File Location"() -> (w411:path)
          n292 = global read "Auto Drive Calibrations.vi" "Auto Drive Calibrations File Location"() -> (w389:path)
          n293 = global read "Shooter Calibrations.vi" "Shooter Calibrations File Location"() -> (w412:path)
          n294 = global read "Ball Intake Calibrations.vi" "Ball Intake Calibrations File Location"() -> (w413:path)
          n295 = Greater Or Equal?(x=w432, y=5) -> (x >= y?=w430:bool)
          n296 = global read "Drive Path Calibrations.vi" "Drive Path Calibrations File Location"() -> (w401:path)
          n297 = Array To Spreadsheet String(delimiter (Tab)=",", array=w395, 3:"%f" ("format string")) -> (spreadsheet string=w399:string)
          n298 = Array To Spreadsheet String(delimiter (Tab)=",", array=w410, 3:"%f" ("format string")) -> (spreadsheet string=w433:string)
          n299 = Array To Spreadsheet String(delimiter (Tab)=",", array=w400, 3:"%f" ("format string")) -> (spreadsheet string=w404:string)
          n300 = Array To Spreadsheet String(delimiter (Tab)=",", array=w388, 3:"%f" ("format string")) -> (spreadsheet string=w392:string)
          n301 = Array To Spreadsheet String(delimiter (Tab)=",", array=w408, 3:"%f" ("format string")) -> (spreadsheet string=w423:string)
          n302 = Array To Spreadsheet String(delimiter (Tab)=",", array=w407, 3:"%f" ("format string")) -> (spreadsheet string=w414:string)
          n303 = Array To Spreadsheet String(delimiter (Tab)=",", array=w406, 3:"%f" ("format string")) -> (spreadsheet string=w417:string)
          n304 = Array To Spreadsheet String(delimiter (Tab)=",", array=w405, 3:"%f" ("format string")) -> (spreadsheet string=w420:string)
          n305 = Array To Spreadsheet String(delimiter (Tab)=",", array=w409, 3:"%f" ("format string")) -> (spreadsheet string=w426:string)
          n306 = Write to Text File(file (use dialog)=w429, text=w433) -> ()  [unwired: 2 in, 3 out]
          n307 = Write to Text File(file (use dialog)=w396, text=w399) -> ()  [unwired: 2 in, 3 out]
          n308 = Write to Text File(file (use dialog)=w401, text=w404) -> ()  [unwired: 2 in, 3 out]
          n309 = Write to Text File(file (use dialog)=w389, text=w392) -> ()  [unwired: 2 in, 3 out]
          n310 = Write to Text File(file (use dialog)=w394, text=w423) -> ()  [unwired: 2 in, 3 out]
          n311 = Write to Text File(file (use dialog)=w413, text=w414) -> ()  [unwired: 2 in, 3 out]
          n312 = Write to Text File(file (use dialog)=w412, text=w417) -> ()  [unwired: 2 in, 3 out]
          n313 = Write to Text File(file (use dialog)=w411, text=w420) -> ()  [unwired: 2 in, 3 out]
          n314 = Write to Text File(file (use dialog)=w393, text=w426) -> ()  [unwired: 2 in, 3 out]
        }
        n315 = Select(t=w386, s=w385, f=u32 2) -> (s? t:f=w383:u32)
      }
    }
    n316 = feedback-in #2(w145) -> ()
  }
